vi "平行样启动参数选择对话框.vi"() -> (1 "取消启动":bool, 2 "确定启动":bool, 3 "启动模块":cluster{"氨氮1":bool, "总磷1":bool, " COD1":bool})   [LabVIEW 2016, in "质控单元.lvlib"]
panel:
  in  "确定":bool
  in  "COD":bool
  in  "总磷":bool
  in  "取消":bool
  in  "氨氮":bool
  # "请选择平行样测试模块"
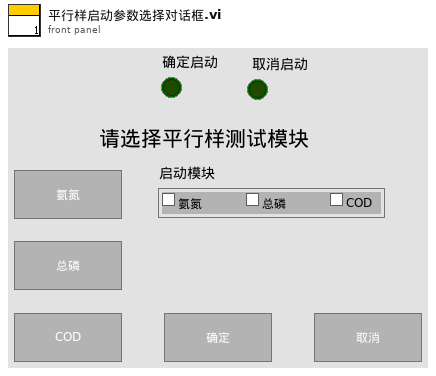
[diagram p1: front panel]
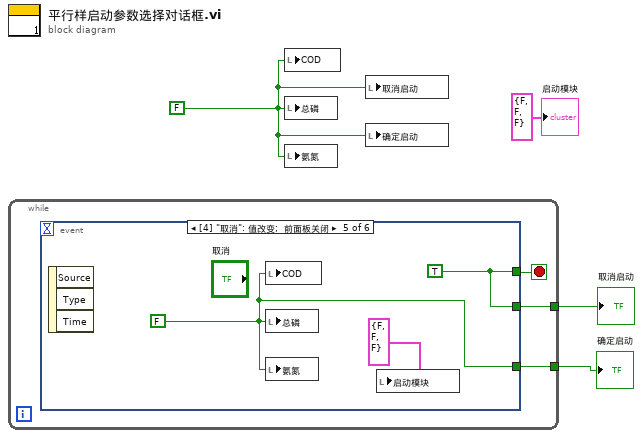
[diagram p0: block diagram]
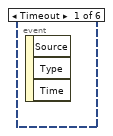
[diagram p2: hidden frame]
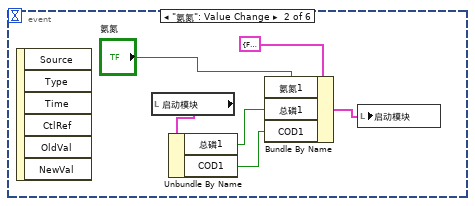
[diagram p3: hidden frame]
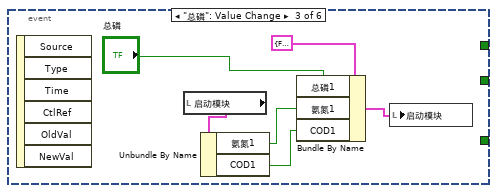
[diagram p4: hidden frame]
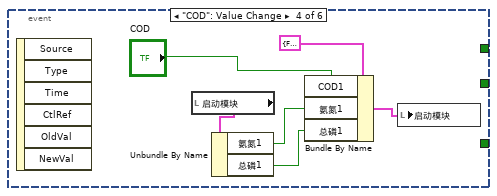
[diagram p5: hidden frame]
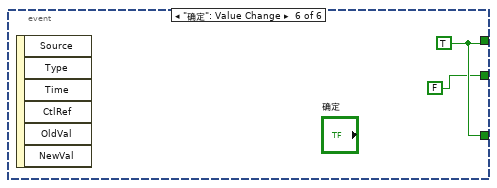
[diagram p6: hidden frame]
diagram:
  w1 = FALSE ("确定")
  n1 = while {
    tunnel: [w6] -> w3
    tunnel: [w5] -> w2
    stop <- w7 stop-if-true
    n2 = event shown="[4] \"取消\": 值改变;  前面板关闭" {
      selector: _ -> [_ _ _ _ _ _]
      dyn-events: _ -> [_ _ _ _ _ _]
      timeout: _ -> [_ _ _ _ _ _]
      tunnel: [_ _ _ _ w27 w30] -> w7
      tunnel: [_ _ _ _ w26 w30] -> w6
      tunnel: [_ _ _ _ w27 FALSE ("确定")] -> w5
      event Timeout {
        n3 = event-data() -> ()  [unwired: 1 in, 3 out]
      }
      event "氨氮": Value Change {
        n4 = event-data() -> ()  [unwired: 1 in, 6 out]
        n5 = local read "启动模块"() -> (w11:cluster{"氨氮1":bool, "总磷1":bool, " COD1":bool})
        n6 = Unbundle By Name(w11) -> ("总磷1"=w10:bool, "COD1"=w9:bool)
        n7 = Bundle By Name(cluster=cluster{"氨氮1":bool, "总磷1":bool, " COD1":bool} {"氨氮1"=FALSE, "总磷1"=FALSE, " COD1"=FALSE} ("启动模块"), "氨氮1"="氨氮", "总磷1"=w10, "COD1"=w9) -> (w8:cluster{"氨氮1":bool, "总磷1":bool, " COD1":bool})
        n8 = local write "启动模块"(w8) -> ()
      }
      event "总磷": Value Change {
        n9 = event-data() -> ()  [unwired: 1 in, 6 out]
        n10 = local read "启动模块"() -> (w18:cluster{"氨氮1":bool, "总磷1":bool, " COD1":bool})
        n11 = Unbundle By Name(w18) -> ("氨氮1"=w17:bool, "COD1"=w16:bool)
        n12 = Bundle By Name(cluster=cluster{"氨氮1":bool, "总磷1":bool, " COD1":bool} {"氨氮1"=FALSE, "总磷1"=FALSE, " COD1"=FALSE} ("启动模块"), "总磷1"="总磷", "氨氮1"=w17, "COD1"=w16) -> (w15:cluster{"氨氮1":bool, "总磷1":bool, " COD1":bool})
        n13 = local write "启动模块"(w15) -> ()
      }
      event "COD": Value Change {
        n14 = event-data() -> ()  [unwired: 1 in, 6 out]
        n15 = local read "启动模块"() -> (w24:cluster{"氨氮1":bool, "总磷1":bool, " COD1":bool})
        n16 = Unbundle By Name(w24) -> ("氨氮1"=w23:bool, "总磷1"=w22:bool)
        n17 = Bundle By Name(cluster=cluster{"氨氮1":bool, "总磷1":bool, " COD1":bool} {"氨氮1"=FALSE, "总磷1"=FALSE, " COD1"=FALSE} ("启动模块"), "COD1"="COD", "氨氮1"=w23, "总磷1"=w22) -> (w21:cluster{"氨氮1":bool, "总磷1":bool, " COD1":bool})
        n18 = local write "启动模块"(w21) -> ()
      }
      event "取消": Value Change; Panel Close {
        w26 = FALSE ("确定")
        w27 = TRUE ("确定")
        n19 = event-data() -> ()  [unwired: 1 in, 3 out]
        n20 = local write "COD"(w26) -> ()
        n21 = local write "总磷"(w26) -> ()
        n22 = local write "氨氮"(w26) -> ()
        n23 = local write "启动模块"(cluster{"氨氮1":bool, "总磷1":bool, " COD1":bool} {"氨氮1"=FALSE, "总磷1"=FALSE, " COD1"=FALSE} ("启动模块")) -> ()
      }
      event "确定": Value Change {
        w30 = TRUE ("确定")
        n24 = event-data() -> ()  [unwired: 1 in, 6 out]
      }
    }
  }
  "确定启动" <- w3
  "取消启动" <- w2
  n25 = local write "COD"(w1) -> ()
  n26 = local write "总磷"(w1) -> ()
  n27 = local write "氨氮"(w1) -> ()
  n28 = local write "取消启动"(w1) -> ()
  n29 = local write "确定启动"(w1) -> ()
  "启动模块" <- cluster{"氨氮1":bool, "总磷1":bool, " COD1":bool} {"氨氮1"=FALSE, "总磷1"=FALSE, " COD1"=FALSE} ("启动模块")
